vi "Impedance_Single.vi"(0 "Test Params Cluster":T4={"Test Freq. (Hz)"=25000.0, "Output Signal Amplitude\nVolts Pk"=0.1, "Sampling Time (s)"=0.01, "Sampling Rate (Hz)"=250000.0, "Output Channel"="PXI1Slot2/ao1", "Current Channel"="PXI1Slot2/ai1", "Voltage Channel"="PXI1Slot2/ai0", "Trigger Channel"="/PXI1Slot2/ao/StartTrigger", "Number of runs"=5}, 2 "SaveFile?":bool, 5 "LCR Params":T3={"Rg_Vmon"=5000.0, "Rg_Imon"=5000.0, "ESL_Cal"=2.95e-07, "ESR_Cal"=0.0, "Cp_Cal"=0.0, "Rp_Cal"=1000000000.0, "UseCorrection"=TRUE, "R_Shunt"=100.0, "RLoad"=1000000000.0, "RLoad_Meas"=1000000000.0} {"RLoad_Meas" format="%#_6p"; "RLoad" format="%#_6p"; "R_Shunt" format="%#_6p"; "Rg_Vmon" format="%#_6p"; "Rg_Imon" format="%#_6p"; "ESL_Cal" format="%#_6p"; "ESR_Cal" format="%#_6p"; "Cp_Cal" format="%#_6p"; "Rp_Cal" format="%#_6p"}, 7 "Saving Cluster":T2={"Experiment Title"="Experiment Title", "Save Path"=path "C:/Users/Human-MPI/Desktop/Temp", "File Name String"="TestStats", "Meta-Data Array"=[]}) -> (1 "Progress":i32(slide) scale=0.0..100.0, 4 "Mean Signal\nImpedance cluster":T5={"|Z|"=131.4492234563314, "Phase(Z)"=77.90762243322018, "Re(Z)"=27.537098036686675, "Imag(Z)"=128.53251175866149, "Ls"=0.0008182633837763256, "Cs"=-4.952986319624157e-08, "Rp"=0.0, "Cp"=0.0} {"|Z|" format="%#_6p"; "Phase(Z)" format="%#_6p"; "Re(Z)" format="%#_6p"; "Imag(Z)" format="%#_6p"; "Ls" format="%#_6p"; "Cs" format="%#_6p"; "Rp" format="%#_6p"; "Cp" format="%#_6p"}, 13 "Debug Cluster":T1 {"VMon-Ampl" format="%.2p"; "IMon-Ampl" format="%.2p"; "THD-VMon" format="%.2p"; "THD-IMon" format="%.2p"; "detected fundamental frequency" format="%.2p"})   [LabVIEW 2021]
uses:
  <vilib>/measure/mascope.llb/Amplitude and Levels 1 chan.vi
  <vilib>/measure/matone.llb/Harmonic Distortion Analyzer 1 Chan.vi
  <vilib>/Analysis/baseanly.llb/Mean (CDB).vi
  <vilib>/Analysis/NI_AALBase.lvlib
  <vilib>/measure/NI_MAPro.lvlib
panel:
  out "Voltage Array":cdb[](array[numeric])
  out "Current Array":cdb[](array[numeric])
  in  "Tab Control":enum32{"Inputs", "Outputs", "Additional Plots"}(tab)
  out "Impedance (Mag)":dbl=131.44922360893165 format="%_4p"
  out "Impedance (Phase)":dbl=77.90762242326527 format="%_3p"
  out "Inductance":dbl=0.0008182633837921632 format="%#_3p"
  out "Capacitance":dbl=-4.9529863304224986e-08 format="%#_3p"
  out "Real (Z)":dbl=27.53709808707976 format="%#_4p"
  out "St. Dev - |Z|":dbl=0.006733204606830156 format="%.4p"
  out "St. Dev - L":dbl=4.20379350558212e-08 format="%.2p"
  out "St. Dev - C":dbl=2.5446531556775277e-12 format="%.2p"
  out "St. Dev - R":dbl=0.00676584259927313 format="%.2p"
  out "Mag Real Imag":cluster{"mean":dbl, "mean":dbl, "Imag(Z)":dbl}(graph)
  out "Time domain Voltage":waveform(dbl)(graph)={"t0"=timestamp(3724414950.391881 s since 1904-01-01), "dt"=3.999999999999989e-06, "Y"=array[2500 elements], "attributes"=variant("NI_ChannelName"=variant(string "Dev3/ai0"), "NI_UnitDescription"=variant(string "Volts"))}
  out "Time domain Current\n(Measured Voltage)":waveform(dbl)(graph)={"t0"=timestamp(3724414950.478328 s since 1904-01-01), "dt"=3.999999999999989e-06, "Y"=array[2500 elements], "attributes"=variant("NI_ChannelName"=variant(string "Dev3/ai1"), "NI_UnitDescription"=variant(string "Volts"))}
  out "Inductance 2":dbl(graph)
  out "Current Run #":i32=4
  out "Time domain Signals":waveform(dbl)[](graph)=[{"t0"=timestamp(3724414950.391881 s since 1904-01-01), "dt"=3.999999999999989e-06, "Y"=array[2500 elements], "attributes"=variant("NI_ChannelName"=variant(string "Dev3/ai0"), "NI_UnitDescription"=variant(string "Volts"))}, {"t0"=timestamp(3724414950.478328 s since 1904-01-01), "dt"=3.999999999999989e-06, "Y"=array[2500 elements], "attributes"=variant("NI_ChannelName"=variant(string "Dev3/ai1"), "NI_UnitDescription"=variant(string "Volts"))}]
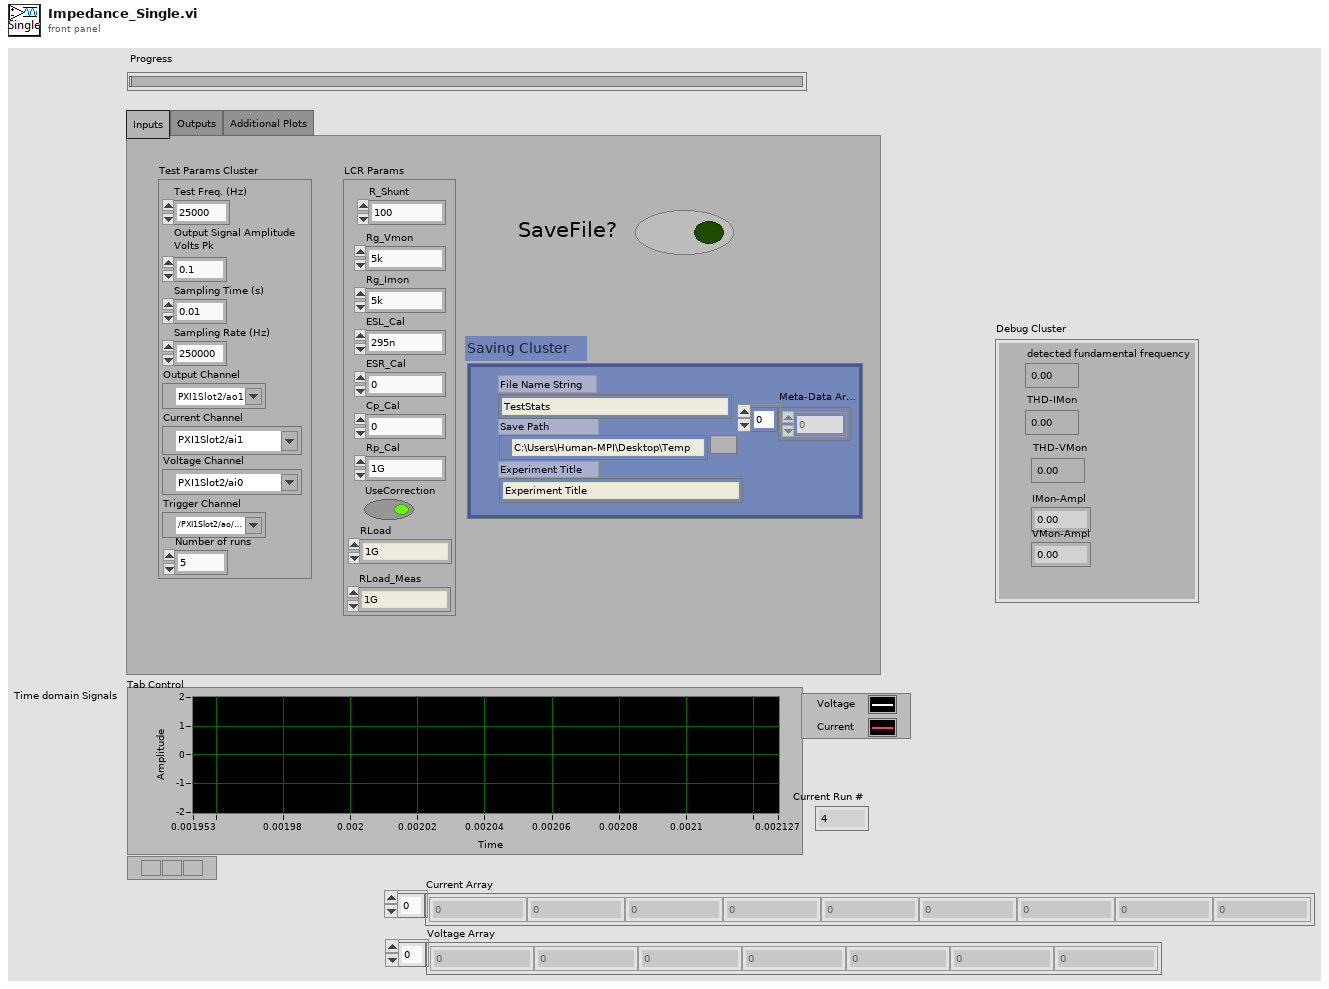
[diagram p1: front panel]
types:
  T1 = cluster{"detected fundamental frequency":dbl, "THD-IMon":dbl, "THD-VMon":dbl, "IMon-Ampl":dbl, "VMon-Ampl":dbl}
  T2 = cluster{"Experiment Title":string, "Save Path":path, "File Name String":string, "Meta-Data Array":dbl[]}
  T3 = cluster{"Rg_Vmon":dbl, "Rg_Imon":dbl, "ESL_Cal":dbl, "ESR_Cal":dbl, "Cp_Cal":dbl, "Rp_Cal":dbl, "UseCorrection":bool, "R_Shunt":dbl, "RLoad":dbl, "RLoad_Meas":dbl}
  T4 = cluster{"Test Freq. (Hz)":dbl, "Output Signal Amplitude\nVolts Pk":dbl, "Sampling Time (s)":dbl, "Sampling Rate (Hz)":dbl, "Output Channel":tag, "Current Channel":tag, "Voltage Channel":tag, "Trigger Channel":tag, "Number of runs":i32}
  T5 = cluster{"|Z|":dbl, "Phase(Z)":dbl, "Re(Z)":dbl, "Imag(Z)":dbl, "Ls":dbl, "Cs":dbl, "Rp":dbl, "Cp":dbl}
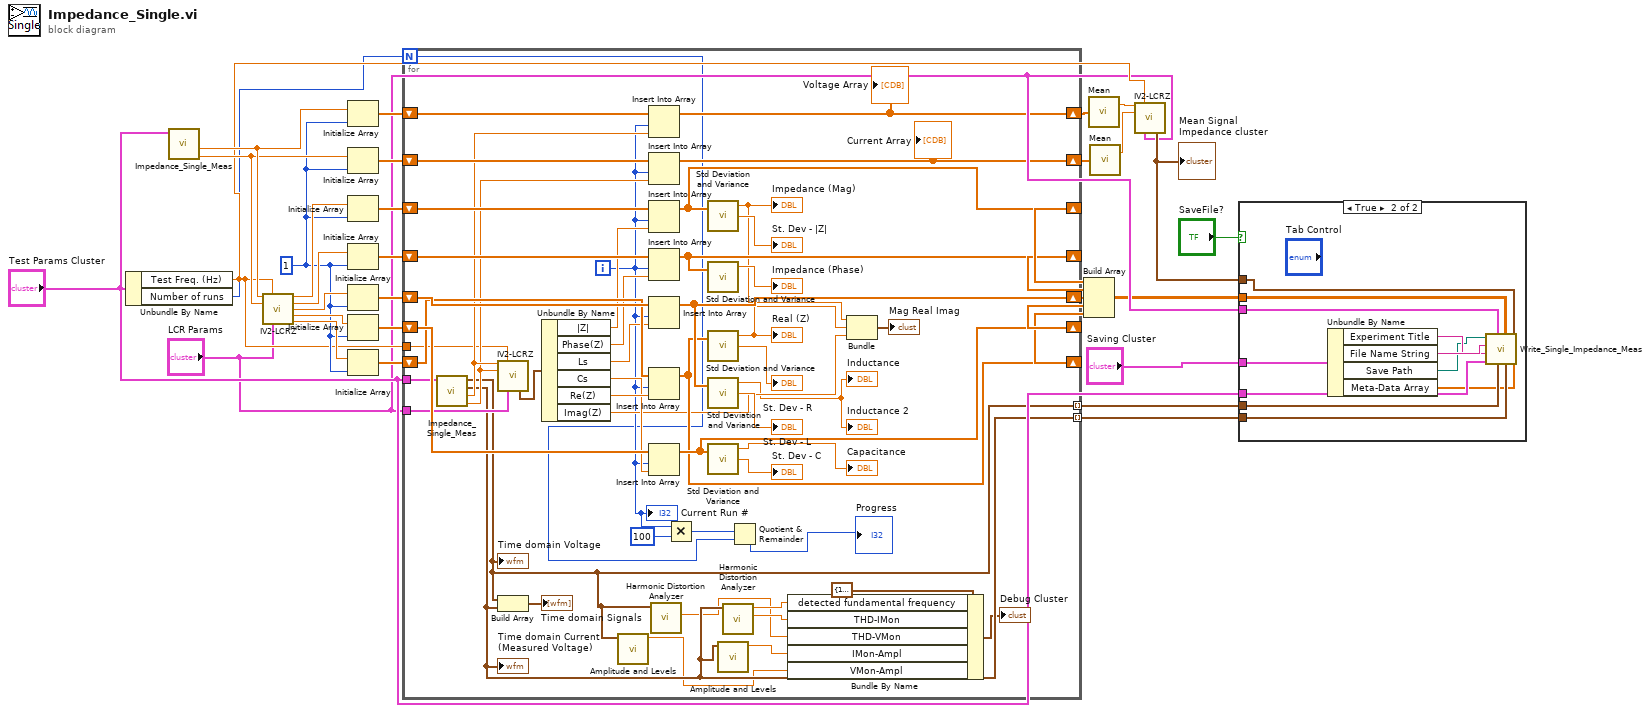
[diagram p0: block diagram]
diagram:
  w22 = 1 ("dimension size")
  n1 = Unbundle By Name("Test Params Cluster") -> ("Test Freq. (Hz)"=w10:dbl, "Number of runs"=w8:i32)
  n2 = call "Impedance_Single_Meas.vi"("Test Params Cluster"="Test Params Cluster") -> ("Current Complex"=w23:cdb, "Voltage Complex"=w24:cdb)  [unwired: 7 in, 2 out]
  n3 = call "IV2-LCRZ.vi"("Voltage In"=w24, "Test Frequency"=w10, "Current In"=w23, "LCR Params"="LCR Params") -> ("Impedance (Mag)"=w32:dbl, "Impedance (Phase)"=w31:dbl, "Ls"=w30:dbl, "Cs"=w29:dbl, "Real (Z)"=w28:dbl)  [unwired: 6 in, 1 out]
  n4 = Initialize Array(w24, w22) -> (w21:cdb[])
  n5 = Initialize Array(w23, w22) -> (w20:cdb[])
  n6 = Initialize Array(w32, w22) -> (w34:dbl[])
  n7 = Initialize Array(w31, w22) -> (w33:dbl[])
  n8 = Initialize Array(w30, w22) -> (w27:dbl[])
  n9 = Initialize Array(w29, w22) -> (w26:dbl[])
  n10 = Initialize Array(w28, w22) -> (w25:dbl[])
  n11 = for {
    N: w8 -> [w44]
    shift-right: [w71] -> w7
    shift-left: w34 -> [w84]
    shift-right: [w70] -> w6
    shift-left: w33 -> [w83]
    shift-right: [w69] -> w5
    shift-left: w27 -> [w82]
    shift-right: [w65] -> w4
    shift-left: w26 -> [w81]
    shift-right: [w63] -> w3
    shift-left: w25 -> [w80]
    shift-right: [w75] -> w19
    shift-left: w21 -> [w79]
    shift-right: [w74] -> w18
    shift-left: w20 -> [w78]
    tunnel: "LCR Params" -> [w62]
    tunnel: "Test Params Cluster" -> [w55]
    tunnel: [w42] -> w13 mode=indexing
    tunnel: [w43] -> w12 mode=indexing
    tunnel: w10 -> [w54]
    i -> [w47]
    n12 = call "Impedance_Single_Meas.vi"("Test Params Cluster"=w55) -> ("Current Complex"=w76:cdb, "Voltage Complex"=w77:cdb, "Time domain Current"=w43:waveform(dbl), "Time domain Voltage"=w42:waveform(dbl))  [unwired: 7 in]
    "Time domain Current\n(Measured Voltage)" <- w43
    "Time domain Voltage" <- w42
    n13 = call "IV2-LCRZ.vi"("Voltage In"=w77, "Test Frequency"=w54, "Current In"=w76, "LCR Params"=w62) -> ("Impedance cluster"=w61:T5)  [unwired: 6 in, 5 out]
    n14 = Build Array(w42, w43) -> (→"Time domain Signals":waveform(dbl)[])
    n15 = Unbundle By Name(w61) -> ("|Z|"=w60:dbl, "Phase(Z)"=w59:dbl, "Ls"=w56:dbl, "Cs"=w57:dbl, "Re(Z)"=w58:dbl, "Imag(Z)"=w50:dbl)
    n16 = call-poly <vilib>:"Amplitude and Levels.vi"("signal in"=w42) -> ("amplitude"=w35:dbl)  [unwired: 7 in, 3 out]
    n17 = Insert Into Array(array=w79, index=w47, new element=w77) -> (w75:cdb[])
    "Voltage Array" <- w75
    n18 = Insert Into Array(array=w78, index=w47, new element=w76) -> (w74:cdb[])
    "Current Array" <- w74
    n19 = Insert Into Array(array=w84, index=w47, new element=w60) -> (w71:dbl[])
    n20 = Insert Into Array(array=w83, index=w47, new element=w59) -> (w70:dbl[])
    n21 = Insert Into Array(array=w82, index=w47, new element=w56) -> (w69:dbl[])
    n22 = Insert Into Array(array=w80, index=w47, new element=w58) -> (w63:dbl[])
    n23 = Insert Into Array(array=w81, index=w47, new element=w57) -> (w65:dbl[])
    n24 = call-poly <vilib>:"Harmonic Distortion Analyzer.vi"("signal in"=w42) -> ("THD"=w37:dbl)  [unwired: 5 in, 5 out]
    n25 = Multiply(x=w47, y=100) -> (x*y=w45:i32)
    n26 = call <vilib>:"Std Deviation and Variance.vi"("X"=w71) -> ("mean"=w52:dbl, "standard deviation"=→"St. Dev - |Z|":dbl)  [unwired: 1 in, 1 out]
    "Impedance (Mag)" <- w52
    n27 = call <vilib>:"Std Deviation and Variance.vi"("X"=w70) -> ("mean"=→"Impedance (Phase)":dbl)  [unwired: 1 in, 2 out]
    n28 = call <vilib>:"Std Deviation and Variance.vi"("X"=w63) -> ("mean"=w51:dbl, "standard deviation"=→"St. Dev - R":dbl)  [unwired: 1 in, 1 out]
    "Real (Z)" <- w51
    n29 = call <vilib>:"Std Deviation and Variance.vi"("X"=w69) -> ("mean"=→"Inductance" →"Inductance 2":dbl, "standard deviation"=→"St. Dev - L":dbl)  [unwired: 1 in, 1 out]
    n30 = call <vilib>:"Std Deviation and Variance.vi"("X"=w65) -> ("mean"=→"Capacitance":dbl, "standard deviation"=→"St. Dev - C":dbl)  [unwired: 1 in, 1 out]
    n31 = call-poly <vilib>:"Amplitude and Levels.vi"("signal in"=w43) -> ("amplitude"=w36:dbl)  [unwired: 7 in, 3 out]
    n32 = call-poly <vilib>:"Harmonic Distortion Analyzer.vi"("signal in"=w43) -> ("THD"=w38:dbl, "detected fundamental frequency"=w40:dbl)  [unwired: 5 in, 4 out]
    n33 = Quotient & Remainder(x=w45, y=w44) -> (floor(x/y)=→"Progress":i32)  [unwired: 1 out]
    n34 = Bundle By Name(cluster=T1 {"detected fundamental frequency"=162562.78926963735, "THD-IMon"=0.006405387428396915, "THD-VMon"=0.0018502712474100448, "IMon-Ampl"=0.821913373414634, "VMon-Ampl"=0.4876277523543882} ("Debug Cluster"), "detected fundamental frequency"=w40, "THD-IMon"=w38, "THD-VMon"=w37, "IMon-Ampl"=w36, "VMon-Ampl"=w35) -> (→"Debug Cluster":T1)
    n35 = Bundle("mean"=w52, "mean"=w51, "Imag(Z)"=w50) -> (→"Mag Real Imag":cluster{"mean":dbl, "mean":dbl, "Imag(Z)":dbl})  [unwired: 1 in]
    "Current Run #" <- w47
  }
  n36 = Build Array(w7, w6, w5, w4, w3) -> (w2:dbl[][])
  n37 = call-poly <vilib>:"Mean.vi"("X"=w19) -> ("mean"=w17:cdb)  [unwired: 1 out]
  n38 = call-poly <vilib>:"Mean.vi"("X"=w18) -> ("mean"=w16:cdb)  [unwired: 1 out]
  n39 = call "IV2-LCRZ.vi"("Voltage In"=w17, "Test Frequency"=w10, "Current In"=w16, "LCR Params"="LCR Params") -> ("Impedance cluster"=w15:T5)  [unwired: 6 in, 5 out]
  "Mean Signal\nImpedance cluster" <- w15
  n40 = case shown="True" "SaveFile?" {
    tunnel: "Test Params Cluster" -> [_ w96]
    tunnel: w15 -> [_ w95]
    tunnel: "LCR Params" -> [_ w94]
    tunnel: w13 -> [_ w93]
    tunnel: w12 -> [_ w92]
    tunnel: w2 -> [_ w91]
    tunnel: "Saving Cluster" -> [_ w90]
    frame False {
    }
    frame True {
      n41 = Unbundle By Name(w90) -> ("Experiment Title"=w88:string, "File Name String"=w89:string, "Save Path"=w87:path, "Meta-Data Array"=w86:dbl[])
      n42 = call "Write_Single_Impedance_Meas.vi"("Meta-Data Array"=w86, "Mean Signal\nImpedance cluster"=w95, "Current"=w92, "Run Impedances array"=w91, "Voltage"=w93, "Compensation and Gain"=w94, "Test Params Cluster"=w96, "Experiment Title"=w88, "File Name String"=w89, "Path"=w87) -> ()  [unwired: 2 in]
    }
  }
